vi "Manual Assembly DB_01102025.vi"() -> ()   [LabVIEW 2021]
uses:
  Classes/Routine/Routine Enum.ctl
  Classes/Assembly/Database Entry/Database Entry.lvclass
  Classes/Assembly/Assembly Run.lvclass
  Classes/Workspace/Fixture Enum.ctl
  <vilib>/Utility/file.llb/Read Delimited Spreadsheet (string).vi
  SubVIs/PUT_region.vi
  SubVIs/component_tray_region.vi
  SubVIs/assembly_tray_region.vi
  Classes/Routine/Routine.lvclass
  Classes/Workspace/Fixture.lvclass
  Classes/Controller/Controller.lvclass
  <vilib>/JDP Science/JDP Science Common Utilities/JDP Utility.lvlib
panel:
  in  "Update comments":bool
  out "Status":string
  out "Stack names":T1
  out "Feet check":bool
  out "Assembly Type":string[](array[string])
  out "Assembly tray region":dbl
  out "Component tray region":dbl
  out "PUT Region":dbl
  in  "Clear All":bool
  in  "Assemble":bool
  in  "Pick and Place":bool
  in  "Dispense glue":bool
  in  "Go":bool
  in  "Routine":T2=enum."Dispense Epoxy"
  in  "Update":bool
  in  "Stage":i32(listbox)=-1
  in  "Stop":bool
  in  "Remove":bool
  in  "Add":bool
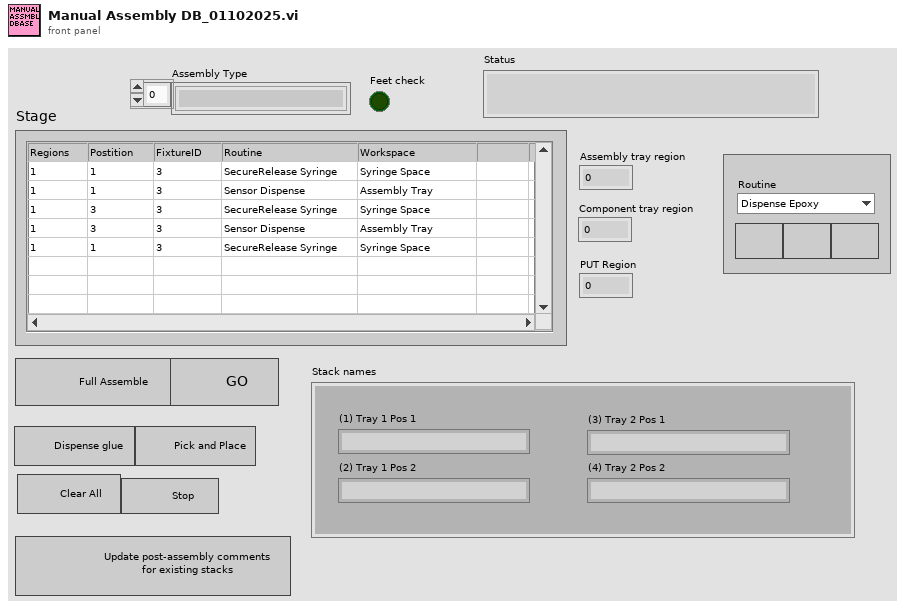
[diagram p1: front panel]
types:
  T1 = cluster{"(1) Tray 1 Pos 1":string, "(2) Tray 1 Pos 2":string, "(3) Tray 2 Pos 1":string, "(4) Tray 2 Pos 2":string}
  T2 = typedef "Routine.lvclass/Routine Enum.ctl" = enum16{"Primary Pick Up", "Secondary Pick Up", "Put Down All", "Secure Syringe", "Release Syringe", "Dispense Epoxy", "Pick Up All", "Put Down Secondary", "Full Assembly"}
  T3 = typedef "Fixture.lvclass/Fixture Enum.ctl" = enum16{"Assembly Tray", "Syringe Space", "Component", "Pick Up Tool", "Current Position"}
  T4 = typedef "File Paths.ctl" = cluster{"Glue Pattern Folder":path, "Carrier Tray Folder":path, "Pick Up Tool Fixture Folder":path, "Components Folder":path, "Bellows Tool Offset.txt":path, "Pick Up Tool Offset.txt":path, "Dispense Tip Offset.txt":path, "Log Files":path, "Gantry Assembly Map.txt":path, "Syringe and offset map.txt":path, "Controllers Folder":path, "Local dbase config":path}
  T5 = cluster{"Fixture ID":dbl, "Position":dbl, "Thickness":dbl}[]
  T6 = cluster{"Stack names[0]":string, "Stack names[1]":string, "Stack names[2]":string, "Stack names[3]":string}
  T7 = typedef "Controller.lvclass/Controllers.ctl" = cluster{"I-O.lvclass":refnum<class "I-O.lvclass">, "Gantry":refnum<k24>, "Dispenser":refnum<visa-resource-name>}
  T8 = cluster{"Fixture ID":dbl, "Position":dbl, "Thickness":dbl}
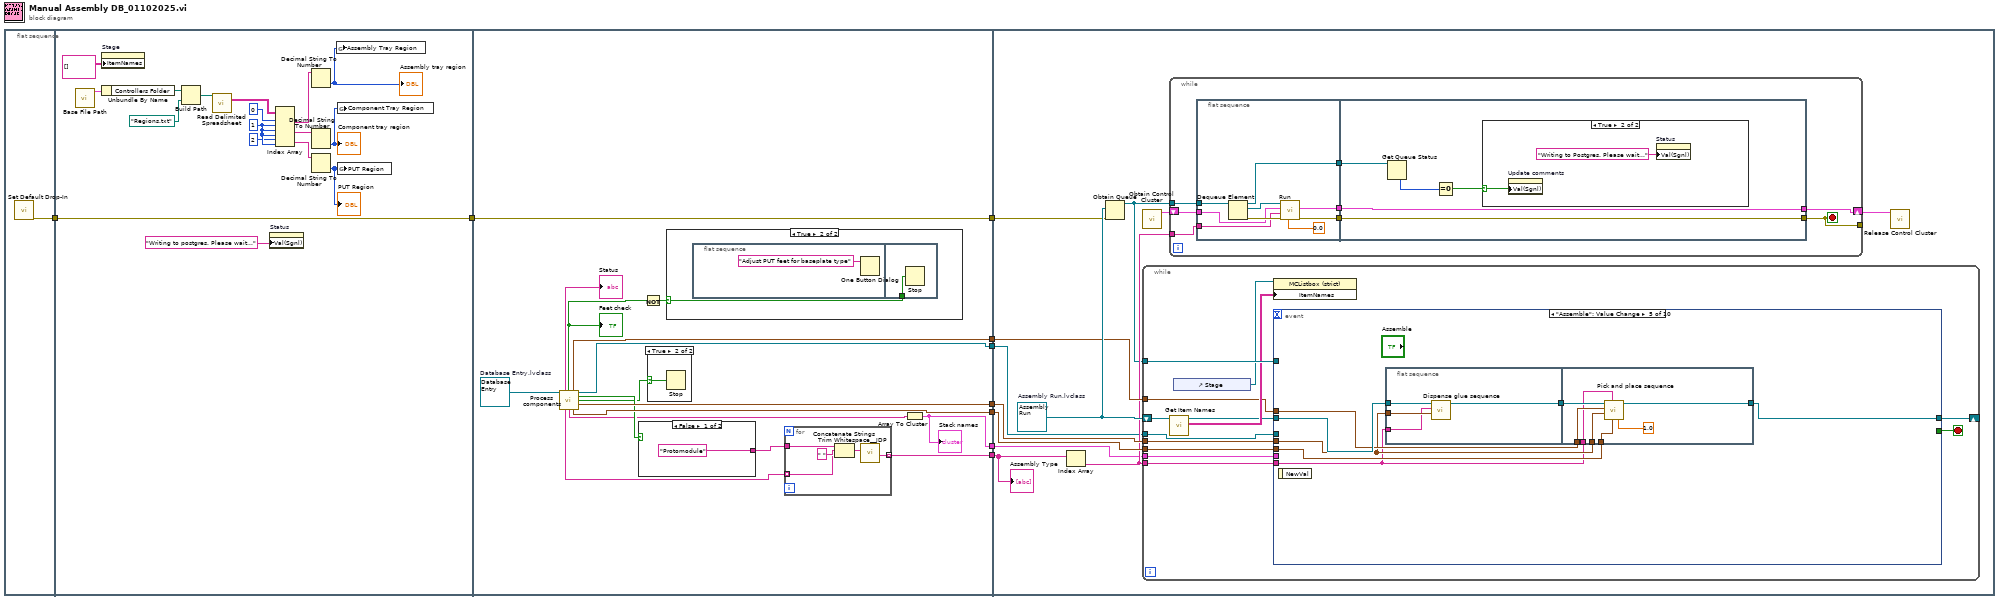
[diagram p0: block diagram]
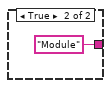
[diagram p4: hidden frame]
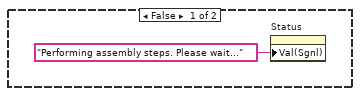
[diagram p5: hidden frame]
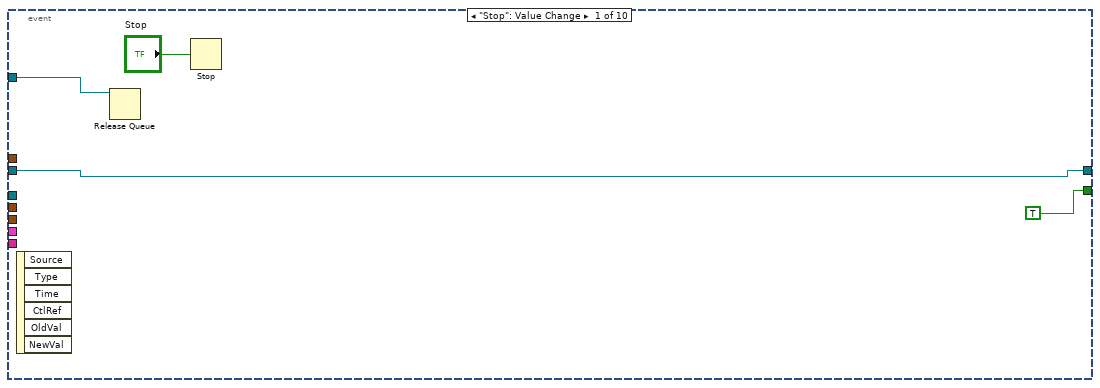
[diagram p6: hidden frame]
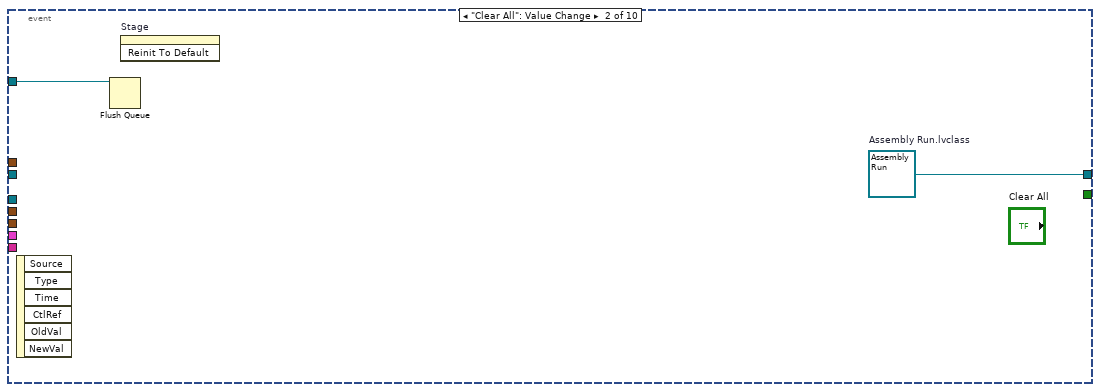
[diagram p7: hidden frame]
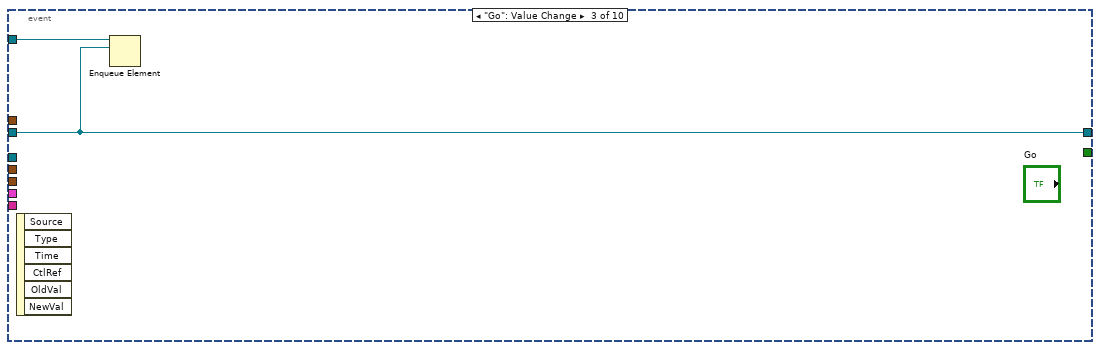
[diagram p8: hidden frame]
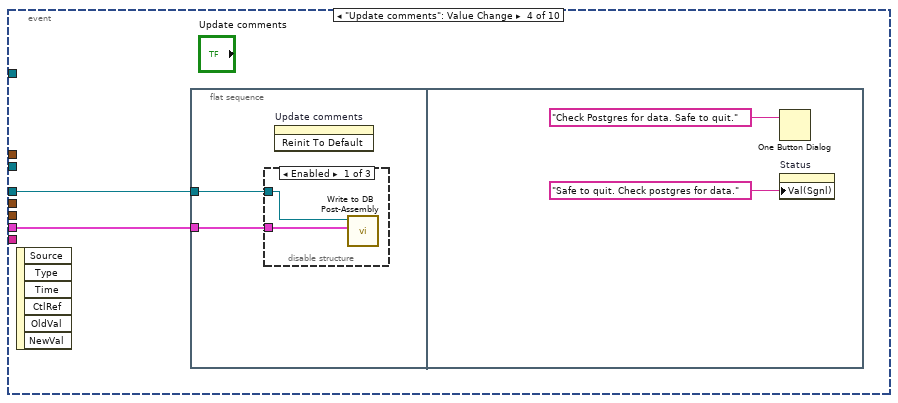
[diagram p9: hidden frame]
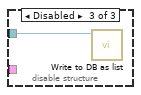
[diagram p11: hidden frame]
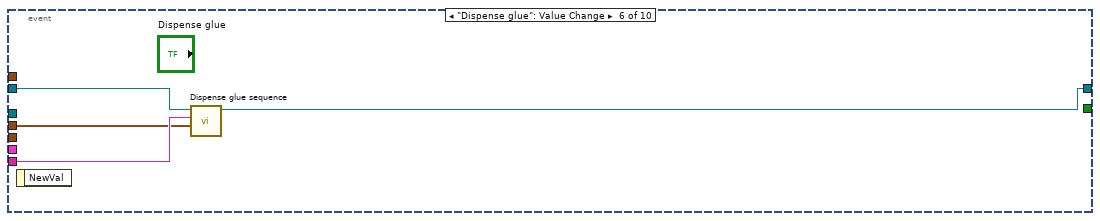
[diagram p12: hidden frame]
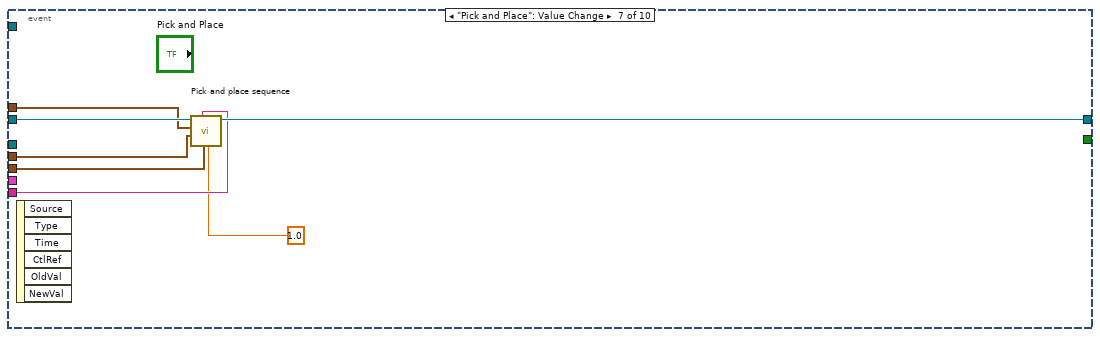
[diagram p13: hidden frame]
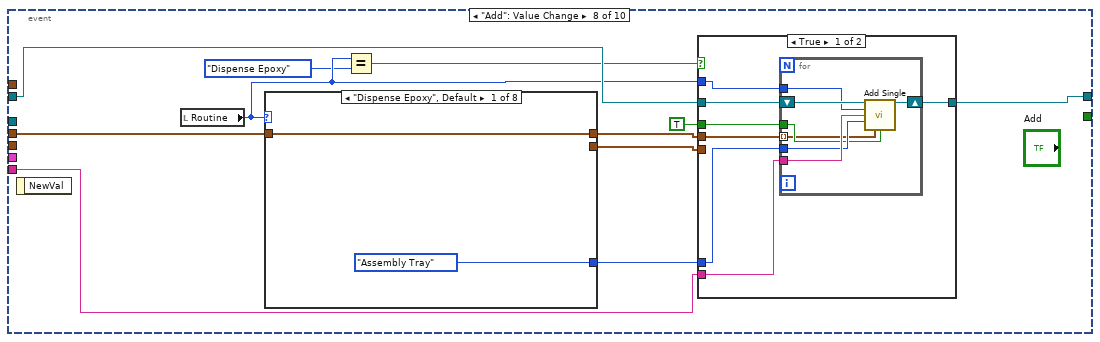
[diagram p14: hidden frame]
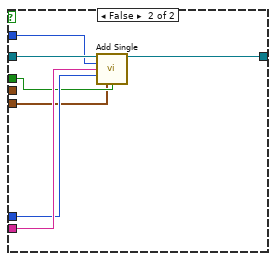
[diagram p15: hidden frame]
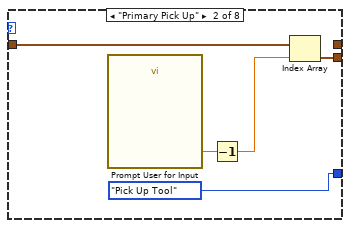
[diagram p16: hidden frame]
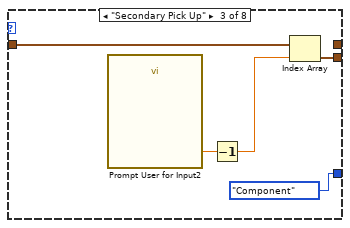
[diagram p17: hidden frame]
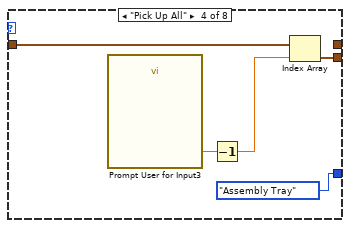
[diagram p18: hidden frame]
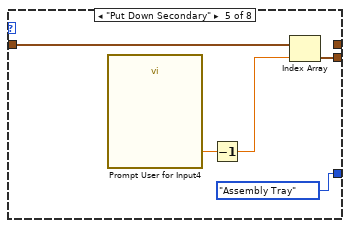
[diagram p19: hidden frame]
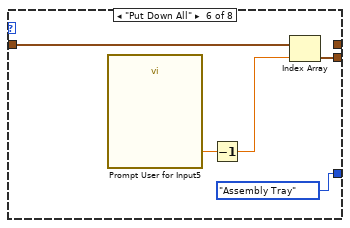
[diagram p20: hidden frame]
diagram:
  n1 = flat-sequence {
    tunnel: [w10] -> w7
    tunnel: [w13] -> w8
    tunnel: w7 -> [w13]
    tunnel: [w42] -> w9
    tunnel: w8 -> [w42]
    tunnel: [w41] -> w6
    tunnel: [w40] -> w5
    tunnel: [w39] -> w4
    tunnel: [w35] -> w3
    tunnel: [w30] -> w2
    tunnel: [w28] -> w1
    tunnel: w9 -> [w65]
    tunnel: w6 -> [w64]
    tunnel: w5 -> [w63]
    tunnel: w4 -> [w62]
    tunnel: w3 -> [w61]
    tunnel: w2 -> [w56]
    tunnel: w1 -> [w57]
    frame #0 {
      n2 = call "Set Default Drop-In.vi"() -> ("error out"=w10:errorcluster)  [unwired: 11 in]
    }
    frame #1 {
      w16 = 1 ("disabled index (col)")
      n3 = call "Base File Path.vi"() -> ("Paths Out"=w27:T4)  [unwired: 11 in]
      n4 = property on="Stage" class="MCListbox (strict)"("ItemNames"=string[][] []) -> ()  [unwired: 2 in, 2 out]
      n5 = Unbundle By Name(w27) -> ("Controllers Folder"=w25:path)
      n6 = Build Path(base path=w25, name or relative path=path "Regions.txt") -> (appended path=w26:path)
      n7 = call-poly <vilib>:"Read Delimited Spreadsheet.vi"("file path (dialog if empty)"=w26) -> ("all rows"=w14:string[][])  [unwired: 9 in, 5 out]
      n8 = property on="Status" class="Str"("Val(Sgnl)"="Writing to postgres. Please wait..." ("Value (Signaling)")) -> ()  [unwired: 2 in, 2 out]
      n9 = Index Array(array=w14, index (row) #1=0 ("index (row)"), index (col) #1=w16, index (row) #2=w16, index (col) #2=w16, index (row) #3=2 ("disabled index (row)"), index (col) #3=w16) -> (element #1=w19:string, element #2=w18:string, element #3=w20:string)
      n10 = Decimal String To Number(string=w19) -> (number=w22:i32)  [unwired: 2 in, 1 out]
      "Assembly tray region" <- w22
      n11 = Decimal String To Number(string=w18) -> (number=w23:i32)  [unwired: 2 in, 1 out]
      "Component tray region" <- w23
      n12 = Decimal String To Number(string=w20) -> (number=w21:i32)  [unwired: 2 in, 1 out]
      "PUT Region" <- w21
      n13 = global write "assembly_tray_region.vi" "Assembly Tray Region"(w22) -> ()
      n14 = global write "component_tray_region.vi" "Component Tray Region"(w23) -> ()
      n15 = global write "PUT_region.vi" "PUT Region"(w21) -> ()
    }
    frame #2 {
      w43 = refnum<class "Database Entry.lvclass"> refnum  # Database Entry.lvclass
      n16 = call "Process components.vi"("Database Entry in"=w43) -> ("Status"=→"Status":string, "Feet check"=w32:bool, "PUT Settings"=w40:T5, "Database Entry out"=w28:refnum<class "Database Entry.lvclass">, "Module?"=w38:bool, "Aborted"=w31:bool, "Assembly Settings"=w39:T5, "Assembly Type"=w37:string[], "Stack names"=w33:string[], "Component Settings"=w41:T5)  [unwired: 4 in, 1 out]
      "Feet check" <- w32
      n17 = case shown="False" w38 {
        tunnel: ["Protomodule" "Module"] -> w36
        frame False {
        }
        frame True {
        }
      }
      n18 = Not(x=w32) -> (.not. x?=w34:bool)
      n19 = case shown="True" w31 {
        selector: w31 -> [_ w44]
        frame False {
        }
        frame True {
          n20 = Stop(stop? (T)=w44) -> ()
        }
      }
      n21 = case shown="True" w34 {
        selector: w34 -> [_ w45]
        frame False {
        }
        frame True {
          n22 = flat-sequence {
            tunnel: w45 -> [w47]
            frame #0 {
              n23 = One Button Dialog(message="Adjust PUT feet for baseplate type") -> ()  [unwired: 1 in, 1 out]
            }
            frame #1 {
              n24 = Stop(stop? (T)=w47) -> ()
            }
          }
        }
      }
      n25 = for {
        tunnel: w37 -> [w50] mode=indexing
        tunnel: w36 -> [w52]
        tunnel: [w48] -> w35 mode=indexing
        n26 = Concatenate Strings(w52, " " ("string"), w50) -> (w49:string)
        n27 = call <vilib>:"Trim Whitespace__JDP.vi"("String in"=w49) -> ("String out"=w48:string)  [unwired: 6 in]
      }
      n28 = Array To Cluster(array=w33) -> (cluster=w30:T6)
      "Stack names" <- w30
    }
    frame #3 {
      w66 = refnum<class "Assembly Run.lvclass"> refnum  # Assembly Run.lvclass
      n29 = Index Array(array=w61) -> (element=w60:string)  [unwired: 1 in]
      n30 = Obtain Queue(element data type=w66, error in (no error)=w65) -> (queue out=w55:refnum<queue>)  [unwired: 3 in, 2 out]
      n31 = call "Obtain Control Cluster.vi"() -> ("Control Out"=w59:T7)  [unwired: 11 in]
      n32 = while {
        shift-right: [w98] -> _
        shift-left: w66 -> [w100]
        tunnel: w55 -> [w103]
        tunnel: w64 -> [w97]
        tunnel: w63 -> [w96]
        tunnel: w62 -> [w95]
        tunnel: w60 -> [w94]
        tunnel: w57 -> [w93]
        tunnel: w56 -> [w92]
        stop <- w104 stop-if-true
        n33 = call "Get Item Names.vi"("Assembly Run in"=w100) -> ("Item names"=w102:string[][], "Assembly Run out"=w99:refnum<class "Assembly Run.lvclass">)  [unwired: 8 in, 1 out]
        n34 = control-ref of="Stage"() -> (w101:refnum<vi>)
        n35 = property class="MCListbox (strict)"(reference=w101, "ItemNames"=w102) -> ()  [unwired: 1 in, 2 out]
        n36 = event shown="[4] \"Assemble\": Value Change" {
          selector: _ -> [_ _ _ _ _ _ _ _ _ _]
          dyn-events: _ -> [_ _ _ _ _ _ _ _ _ _]
          timeout: _ -> [_ _ _ _ _ _ _ _ _ _]
          tunnel: [TRUE _ _ _ _ _ _ _ _ _] -> w104
          tunnel: w99 -> [w107 _ w111 _ w128 w143 w150 w160 w222 w225]
          tunnel: [w107 w110 w111 _ w127 w142 w149 w161 w221 w224] -> w98
          tunnel: w103 -> [w106 w109 w112 _ _ _ _ _ _ _]
          tunnel: w97 -> [_ _ _ _ w124 _ w144 _ _ _]
          tunnel: w96 -> [_ _ _ _ w125 _ w148 _ _ _]
          tunnel: w95 -> [_ _ _ _ w123 w140 w145 w156 w217 _]
          tunnel: w94 -> [_ _ _ _ w122 w141 w147 w159 w218 _]
          tunnel: w93 -> [_ _ _ w114 _ _ _ _ _ _]
          tunnel: w92 -> [_ _ _ w113 _ _ _ _ _ _]
          event "Stop": Value Change {
            n37 = event-data() -> ()  [unwired: 1 in, 6 out]
            n38 = Release Queue(queue=w106) -> ()  [unwired: 2 in, 3 out]
            n39 = Stop(stop? (T)="Stop") -> ()
          }
          event "Clear All": Value Change {
            w110 = refnum<class "Assembly Run.lvclass"> refnum  # Assembly Run.lvclass
            n40 = event-data() -> ()  [unwired: 1 in, 6 out]
            n41 = Flush Queue(queue=w109) -> ()  [unwired: 1 in, 3 out]
            n42 = invoke on="Stage" class="MCListbox (strict)" method="Reinit To Default"() -> ()  [unwired: 3 in, 3 out]
          }
          event "Go": Value Change {
            n43 = event-data() -> ()  [unwired: 1 in, 6 out]
            n44 = Enqueue Element(queue=w112, element=w111) -> ()  [unwired: 2 in, 3 out]
          }
          event "Update comments": Value Change {
            n45 = event-data() -> ()  [unwired: 1 in, 6 out]
            n46 = flat-sequence {
              tunnel: w114 -> [w116]
              tunnel: w113 -> [w115]
              frame #0 {
                n47 = disable-structure shown="Enabled" {
                  disable-tunnel: w116 -> [w118 _ w119]
                  disable-tunnel: w115 -> [w117 _ _]
                  frame Enabled {
                    n48 = call "Write to DB Post-Assembly.vi"("Stack names"=w117, "Database Entry in"=w118) -> ()  [unwired: 8 in, 2 out]
                  }
                  frame Disabled {
                  }
                  frame Disabled {
                    n49 = call "Write to DB as list.vi"("Database Entry in"=w119) -> ()  [unwired: 8 in, 3 out]
                  }
                }
                n50 = invoke on="Update comments" class="Bool (strict)" method="Reinit To Default"() -> ()  [unwired: 3 in, 3 out]
              }
              frame #1 {
                n51 = One Button Dialog(message="Check Postgres for data. Safe to quit.") -> ()  [unwired: 1 in, 1 out]
                n52 = property on="Status" class="Str"("Val(Sgnl)"="Safe to quit. Check postgres for data.") -> ()  [unwired: 2 in, 2 out]
              }
            }
          }
          event "Assemble": Value Change {
            n53 = event-data() -> ()  [unwired: 1 in, 1 out]
            n54 = flat-sequence {
              tunnel: [w131] -> w126
              tunnel: w128 -> [w132]
              tunnel: w123 -> [w130]
              tunnel: w122 -> [w129]
              tunnel: [w138] -> w127
              tunnel: w126 -> [w139]
              tunnel: w123 -> [w137]
              tunnel: w125 -> [w136]
              tunnel: w124 -> [w135]
              tunnel: w122 -> [w134]
              frame #0 {
                n55 = call "Dispense glue sequence.vi"("Assembly Tray Settings Array"=w130, "Assembly Type"=w129, "Assembly Run in"=w132) -> ("Assembly Run out"=w131:refnum<class "Assembly Run.lvclass">)  [unwired: 7 in, 1 out]
              }
              frame #1 {
                n56 = call "Pick and place sequence.vi"("Numeric"=1.0, "Component Tray map"=w135, "Assembly Type"=w134, "Assembly Tray map"=w137, "PUT map"=w136, "Assembly Run in"=w139) -> ("Assembly Run out"=w138:refnum<class "Assembly Run.lvclass">)  [unwired: 4 in, 1 out]
              }
            }
          }
          event "Dispense glue": Value Change {
            n57 = event-data() -> ()  [unwired: 1 in, 1 out]
            n58 = call "Dispense glue sequence.vi"("Assembly Tray Settings Array"=w140, "Assembly Type"=w141, "Assembly Run in"=w143) -> ("Assembly Run out"=w142:refnum<class "Assembly Run.lvclass">)  [unwired: 7 in, 1 out]
          }
          event "Pick and Place": Value Change {
            n59 = event-data() -> ()  [unwired: 1 in, 6 out]
            n60 = call "Pick and place sequence.vi"("Numeric"=1.0, "Component Tray map"=w144, "Assembly Type"=w147, "Assembly Tray map"=w145, "PUT map"=w148, "Assembly Run in"=w150) -> ("Assembly Run out"=w149:refnum<class "Assembly Run.lvclass">)  [unwired: 4 in, 1 out]
          }
          event "Add": Value Change {
            n61 = event-data() -> ()  [unwired: 1 in, 1 out]
            n62 = local read "Routine"() -> (w154:T2)
            n63 = case shown="\"Dispense Epoxy\", Default" w154 {
              tunnel: [Fixture_Enum."Assembly Tray" ("Fixture") Fixture_Enum."Pick Up Tool" ("Fixture") Fixture_Enum."Component" ("Fixture") Fixture_Enum."Assembly Tray" ("Fixture") Fixture_Enum."Assembly Tray" ("Fixture") Fixture_Enum."Assembly Tray" ("Fixture") Fixture_Enum."Syringe Space" ("Fixture") Fixture_Enum."Syringe Space" ("Fixture")] -> w158
              tunnel: w156 -> [w183 w188 w191 w196 w201 w205 w211 w214]
              tunnel: [_ w185 w190 w195 w200 w206 w210 w213] -> w151
              tunnel: [w183 _ _ _ _ _ _ _] -> w152
              frame "Dispense Epoxy", Default {
              }
              frame "Primary Pick Up" {
                n64 = call "Prompt User for Input"() -> ("Position"=w187:dbl)  [unwired: 17 in, 2 out]
                n65 = Decrement(x=w187) -> (x-1=w186:dbl)
                n66 = Index Array(array=w188, index=w186) -> (element=w185:T8)
              }
              frame "Secondary Pick Up" {
                n67 = call "Prompt User for Input2"() -> ("Position"=w193:dbl)  [unwired: 17 in, 2 out]
                n68 = Decrement(x=w193) -> (x-1=w192:dbl)
                n69 = Index Array(array=w191, index=w192) -> (element=w190:T8)
              }
              frame "Pick Up All" {
                n70 = call "Prompt User for Input3"() -> ("Position"=w198:dbl)  [unwired: 17 in, 2 out]
                n71 = Decrement(x=w198) -> (x-1=w197:dbl)
                n72 = Index Array(array=w196, index=w197) -> (element=w195:T8)
              }
              frame "Put Down Secondary" {
                n73 = call "Prompt User for Input4"() -> ("Position"=w203:dbl)  [unwired: 17 in, 2 out]
                n74 = Decrement(x=w203) -> (x-1=w202:dbl)
                n75 = Index Array(array=w201, index=w202) -> (element=w200:T8)
              }
              frame "Put Down All" {
                n76 = call "Prompt User for Input5"() -> ("Position"=w208:dbl)  [unwired: 17 in, 2 out]
                n77 = Decrement(x=w208) -> (x-1=w207:dbl)
                n78 = Index Array(array=w205, index=w207) -> (element=w206:T8)
              }
              frame "Secure Syringe" {
                n79 = Index Array(array=w211) -> (element=w210:T8)  [unwired: 1 in]
              }
              frame "Release Syringe" {
                n80 = Index Array(array=w214) -> (element=w213:T8)  [unwired: 1 in]
              }
            }
            n81 = Equal?(x=w154, y=Routine_Enum."Dispense Epoxy") -> (x = y?=w155:bool)
            n82 = case shown="True" w155 {
              tunnel: [w168 w182] -> w161
              tunnel: w160 -> [w167 w181]
              tunnel: w159 -> [w166 w180]
              tunnel: w158 -> [w165 w179]
              tunnel: w154 -> [w164 w178]
              tunnel: TRUE ("Auto") -> [w163 w177]
              tunnel: w152 -> [w162 _]
              tunnel: w151 -> [_ w176]
              frame True {
                n83 = for {
                  tunnel: w166 -> [w173]
                  tunnel: w165 -> [w172]
                  tunnel: w164 -> [w171]
                  tunnel: w163 -> [w170]
                  shift-right: [w175] -> w168
                  shift-left: w167 -> [w174]
                  tunnel: w162 -> [w169] mode=indexing
                  n84 = call-dynamic "Add Single.vi"("UI in"=w174, "Routine"=w171, "Assembly Type"=w173, "Fixture"=w172, "Input Settings"=w169, "Auto"=w170) -> ("UI out"=w175:refnum<class "Assembly Run.lvclass">)  [unwired: 8 in, 1 out]
                }
              }
              frame False {
                n85 = call-dynamic "Add Single.vi"("UI in"=w181, "Routine"=w178, "Assembly Type"=w180, "Fixture"=w179, "Input Settings"=w176, "Auto"=w177) -> ("UI out"=w182:refnum<class "Assembly Run.lvclass">)  [unwired: 8 in, 1 out]
              }
            }
          }
          event "Update": Value Change {
            n86 = event-data() -> ()  [unwired: 1 in, 6 out]
            n87 = Index Array(array=w217) -> (element=w216:T8)  [unwired: 1 in]
            n88 = call "Update.vi"("Input Settings"=w216, "Assembly Type"=w218, "Row"="Stage", "Routine"="Routine", "Assembly Run in"=w222) -> ("Assembly Run out"=w221:refnum<class "Assembly Run.lvclass">)  [unwired: 5 in, 1 out]
          }
          event "Remove": Value Change {
            n89 = event-data() -> ()  [unwired: 1 in, 6 out]
            n90 = local read "Stage"() -> (w223:i32)
            n91 = call "Delete.vi"("Index"=w223, "Assembly In"=w225) -> ("Assembly Out"=w224:refnum<class "Assembly Run.lvclass">)  [unwired: 8 in, 1 out]
          }
        }
      }
      n92 = while {
        shift-right: [w73] -> w58
        shift-left: w59 -> [w74]
        tunnel: w60 -> [w72]
        tunnel: [w71] -> _
        tunnel: w55 -> [w70]
        stop <- w71 stop-if-true
        n93 = flat-sequence {
          tunnel: w74 -> [w81]
          tunnel: w72 -> [w79]
          tunnel: w70 -> [w76]
          tunnel: [w80] -> w69
          tunnel: [w78] -> w68
          tunnel: [w77] -> w67
          tunnel: [w87] -> w71
          tunnel: [w88] -> w73
          tunnel: w69 -> [w88]
          tunnel: w68 -> [w87]
          tunnel: w67 -> [w86]
          frame #0 {
            n94 = Dequeue Element(queue=w76) -> (queue out=w77:refnum<queue>, element=w83:refnum<class "Assembly Run.lvclass">, error out=w82:errorcluster)  [unwired: 2 in, 1 out]
            n95 = call-dynamic "Run.vi"("Pickup_Test_Number"=0.0, "error in (no error)"=w82, "Assembly Type"=w79, "Control In"=w81, "Assembly In"=w83) -> ("error out"=w78:errorcluster, "Control Out"=w80:T7)  [unwired: 4 in, 1 out]
          }
          frame #1 {
            n96 = Get Queue Status(queue=w86) -> (# elements in queue=w85:i32)  [unwired: 2 in, 7 out]
            n97 = Equal To 0?(x=w85) -> (x = 0?=w84:bool)
            n98 = case shown="True" w84 {
              selector: w84 -> [_ w91]
              frame False {
                n99 = property on="Status" class="Str"("Val(Sgnl)"="Performing assembly steps. Please wait...") -> ()  [unwired: 2 in, 2 out]
              }
              frame True {
                n100 = property on="Update comments" class="Bool (strict)"("Val(Sgnl)"=w91) -> ()  [unwired: 2 in, 2 out]
                n101 = property on="Status" class="Str"("Val(Sgnl)"="Writing to Postgres. Please wait...") -> ()  [unwired: 2 in, 2 out]
              }
            }
          }
        }
      }
      n102 = call "Release Control Cluster.vi"("output cluster"=w58) -> ()  [unwired: 11 in]
      "Assembly Type" <- w61
    }
  }
